vi "Test Parse lvproj with Virtual Folders.vi"(11 "Test Case In":refnum<class "Parsing XML.lvclass">) -> (0 "error out":errorcluster, 3 "Test Case Out":refnum<class "Parsing XML.lvclass">)   [LabVIEW 2020, in "Parsing XML.lvclass"]
uses:
  Parsing XML.lvclass
  source/Classes/Item/Item.lvclass
  Parsing XML.lvclass/Parsing XML.ctl
  4993e8ee-a06a-463a-9684-69129f64d5ce.vi
  source/VI Properties Editor.lvlib
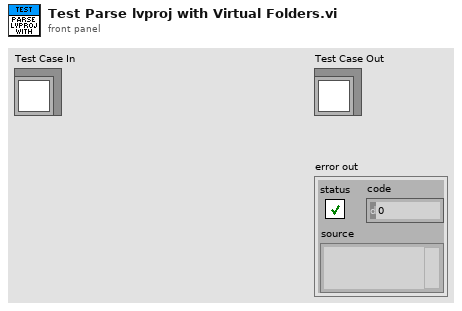
[diagram p1: front panel]
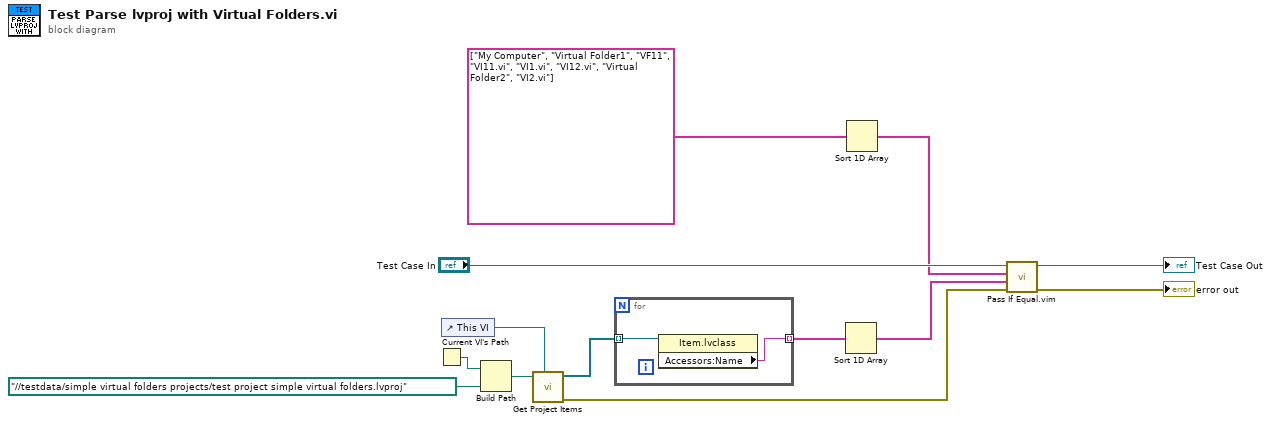
[diagram p0: block diagram]
diagram:
  n1 = Current VI's Path() -> (path=w10:path)
  n2 = control-ref of="This VI"() -> (w1:refnum<vi>)
  n3 = Build Path(base path=w10, name or relative path=path "../../testdata/simple virtual folders projects/test project simple virtual folders.lvproj") -> (appended path=w6:path)
  n4 = call "Get Project Items.vi"("Calling VI Ref"=w1, "Path"=w6) -> ("error out"=w9:errorcluster, "Items Data"=w8:refnum<class "Item.lvclass">[])  [unwired: 7 in, 1 out]
  n5 = for {
    tunnel: w8 -> [w15] mode=indexing
    tunnel: [w14] -> w3 mode=indexing
    n6 = property class="Item.lvclass"(reference=w15) -> ("Accessors:Name"=w14:string)  [unwired: 1 in, 2 out]
  }
  n7 = Sort 1D Array(array=w3) -> (sorted array=w4:string[])
  n8 = Sort 1D Array(array=string[] ["My Computer", "Virtual Folder1", "VF11", "VI11.vi", "VI1.vi", "VI12.vi", "Virtual Folder2", "VI2.vi"] ("Array")) -> (sorted array=w5:string[])
  n9 = call "Pass If Equal.vim"("error in (no error)"=w9, "Actual"=w4, "Expected"=w5, "LUnit Test Case In"="Test Case In") -> ("error out"=→"error out":errorcluster, "LUnit Test Case Out"=→"Test Case Out":refnum<class "Parsing XML.lvclass">)  [unwired: 6 in]
